vi "State_Machine.vi"(8 "error in (no error)":errorcluster caption="entrée d'erreur (pas d'erreur)", 11 "Get_Voltage en entrée":refnum<class "Nodon_Set_Fil_Pilote.lvclass">) -> (0 "error out":errorcluster caption="sortie d'erreur", 2 "Json_String":string, 3 "Get_Voltage en sortie":refnum<class "Nodon_Set_Fil_Pilote.lvclass">)   [LabVIEW 2020, in "Library Test.lvlib" / "Nodon_Set_Fil_Pilote.lvclass"]
uses:
  Nodon_Set_Fil_Pilote.lvclass
  C:/Users/ngarcin/OneDrive - Altyor/Standard TB/Class/Test/Test (Default)/Test (Default).lvclass
  C:/Users/ngarcin/OneDrive - Altyor/Standard TB/Class/Test/Nodon_Send_Command_UART/Nodon_Send_Command_UART.lvclass
  JSON API/JSON Value/Set from JSON string.vi
  JSON API/JSON Value/JSON Value.lvclass
  Nodon_Send_Command_UART.lvclass
  Nodon_Set_Fil_Pilote.lvclass/Nodon_Set_Fil_Pilote.ctl
  JSON API/Variant JSON/Variant JSON.lvlib
  JSON API/Get Polymorphic/JSON GetSet.lvlib
  Commun VI/Library Commun.lvlib
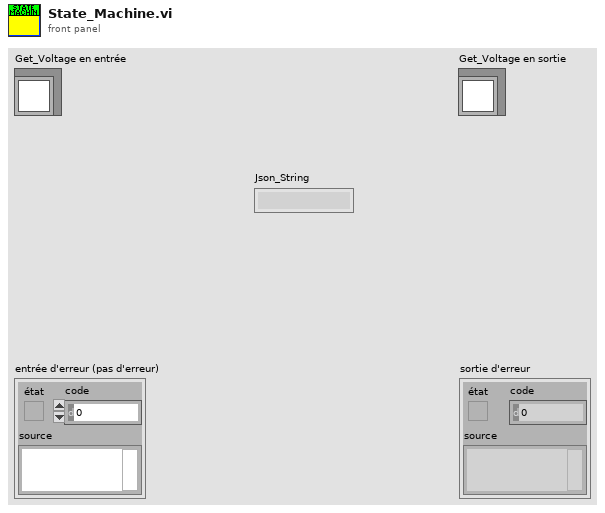
[diagram p1: front panel]
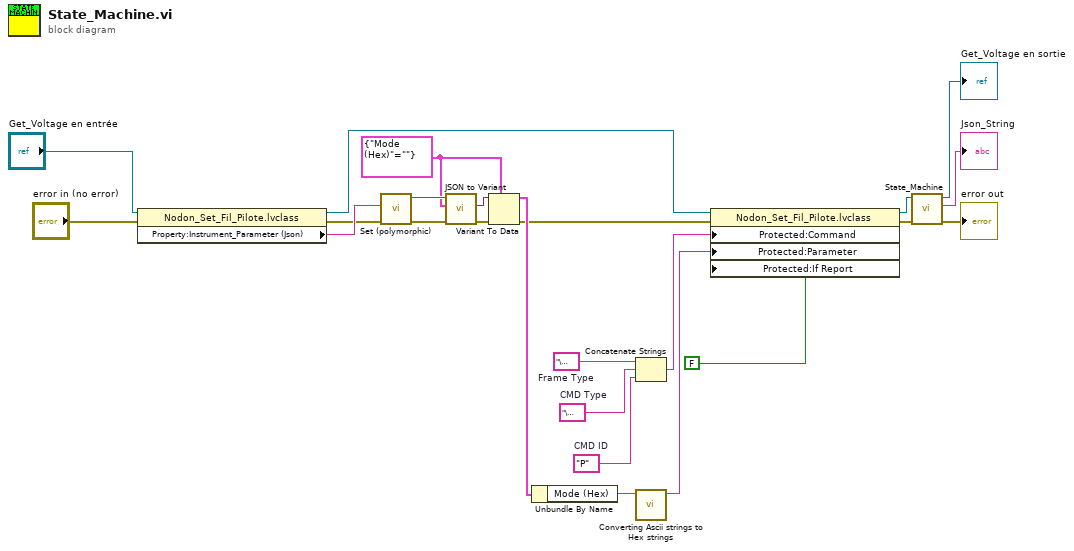
[diagram p0: block diagram]
diagram:
  w8 = cluster{"Mode (Hex)":string} {"Mode (Hex)"=""}
  w19 = "\u0000"  # Frame Type
  w18 = "P"  # CMD ID
  w17 = "\u0000"  # CMD Type
  n1 = property class="Nodon_Set_Fil_Pilote.lvclass"(reference="Get_Voltage en entrée", error in="error in (no error)") -> (reference out=w4:refnum<class "Nodon_Set_Fil_Pilote.lvclass">, error out=w10:errorcluster, "Property:Instrument_Parameter (Json)"=w11:string)
  n2 = call-poly "Set (polymorphic).vi"("error in (no error)"=w10, "JSON stream"=w11) -> ("error out"=w13:errorcluster, "JSON Value out"=w15:refnum<class "JSON Value.lvclass">)  [unwired: 7 in, 1 out]
  n3 = call "JSON to Variant.vi"("error in (no error)"=w13, "Variant (Data Type)"=w8, "JSON Value"=w15) -> ("error out"=w14:errorcluster, "Variant out"=w12:variant)  [unwired: 7 in]
  n4 = Variant To Data(error in=w14, type=w8, Variant=w12) -> (data=w7:cluster{"Mode (Hex)":string}, error out=w6:errorcluster)
  n5 = Unbundle By Name(w7) -> ("Mode (Hex)"=w2:string)
  n6 = Concatenate Strings(w19, w17, w18) -> (w16:string)
  n7 = call "Converting Ascii strings to Hex strings.vi"("result string"=w2) -> ("Chaîne"=w1:string)  [unwired: 10 in]
  n8 = property class="Nodon_Set_Fil_Pilote.lvclass"(reference=w4, error in=w6, "Protected:Command"=w16, "Protected:Parameter"=w1, "Protected:If Report"=FALSE ("If Report")) -> (reference out=w21:refnum<class "Nodon_Set_Fil_Pilote.lvclass">, error out=w20:errorcluster)
  n9 = call-parent "State_Machine.vi"("error in (no error)"=w20, "Send_Frame en entrée"=w21) -> ("error out"=→"error out":errorcluster, "Json_String"=→"Json_String":string, "Send_Frame en sortie"=→"Get_Voltage en sortie":refnum<class "Nodon_Set_Fil_Pilote.lvclass">)  [unwired: 7 in]
